vi "Find USB VISA Names.vi"(11 "error in":errorcluster) -> (4 "VISA names found":string[](array[string]), 15 "error out":errorcluster)   [LabVIEW 2017]
uses:
  <vilib>/Instr/_visa.llb/VISA Find Search Mode.ctl
panel:
  in  "Search Mode":T1=2 items=["Canonical Names Only"=0, "Aliases Only"=2, "Include Matching Aliases"=3, "Include All Aliases"=4]
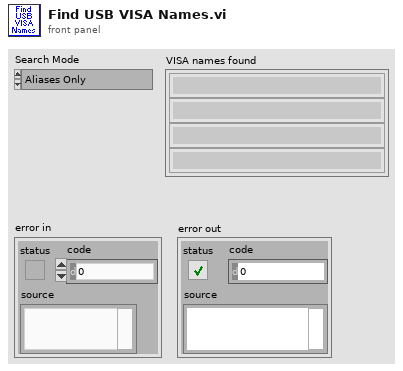
[diagram p1: front panel]
types:
  T1 = typedef "VISA Find Search Mode.ctl" = u32
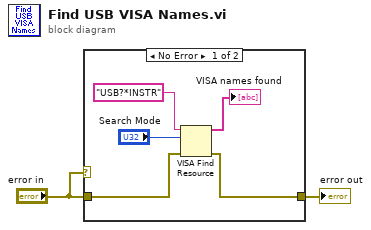
[diagram p0: block diagram]
diagram:
  n1 = case shown="No Error" "error in" {
    tunnel: "error in" -> [w5 w8]
    tunnel: [w3 w8] -> w2
    frame No Error {
      n2 = VISA Find Resource(8:w5, 10:"Search Mode", 11:"USB?*INSTR" ("expression (\"?*\")")) -> (0:w3:errorcluster, 3:→"VISA names found":string[])  [unwired: 1 out]
    }
    frame Error {
    }
  }
  "error out" <- w2
